vi "Test-DotNet-sendLaunchJob.vi"() -> ()   [LabVIEW 2013, in "EC1000-control.lvlib" / "SM1000-control.lvclass"]
uses:
  SM1000-control.lvclass
  DOTNET-settings.ctl
  Device-identification.ctl
  TCP-settings.ctl
panel:
  out "Ready":bool
  out "Job data":string
  out "Elapsed time":dbl caption="Elapsed time [ms]" format="%.2f"
  in  "Abort":bool
  out "Job busy":bool
  in  "Start job":bool
  in  "TCP settings":T1={"Target IP"="128.178.146.163", "Target TCP port"=12500, "TCP read mode"=enum."CRLF", "TCP read buffer"=4096, "Read timeout"=5000}
  in  "Job file path (.xml)":path=path "C:/LabVIEW/TJ-TransferJobs/SampleTestJobs/SM1000-Sim07.xml"
  in  "Device index":i32
  in  "DOTNET settings":T2={"Target IP"="128.178.146.163", "Target broadcast port"=11000, "Target communication port"=12200, "clientID"=-1, "Broadcast IP"="224.168.100.2", "Servercount"=-1, "Device IDs"=[{"Name"="EC1000", "IP"="128.178.146.163", "Mac address"="mac"}]}
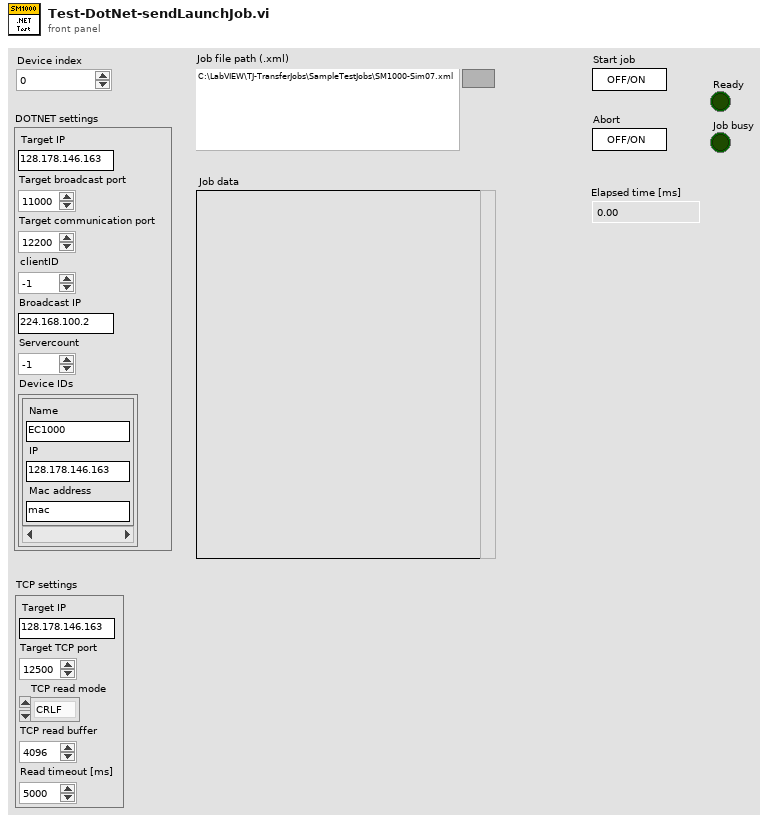
[diagram p1: front panel]
types:
  T1 = typedef "EC1000-control.lvlib/SM1000-control.lvclass/TCP-settings.ctl" = cluster{"Target IP":string, "Target TCP port":u16, "TCP read mode":enum16{"Standard", "Buffered", "CRLF", "Immediate"}, "TCP read buffer":i32, "Read timeout":i32}
  T2 = typedef "EC1000-control.lvlib/SM1000-control.lvclass/DOTNET-settings.ctl" = cluster{"Target IP":string, "Target broadcast port":i32, "Target communication port":i32, "clientID":i32, "Broadcast IP":string, "Servercount":i32, "Device IDs":T3[]}
  T3 = typedef "EC1000-control.lvlib/SM1000-control.lvclass/Device-identification.ctl" = cluster{"Name":string, "IP":string, "Mac address":string}
  T4 = typedef "EC1000-control.lvlib/SM1000-control.lvclass/Object-reference.ctl" = refnum<data-value>
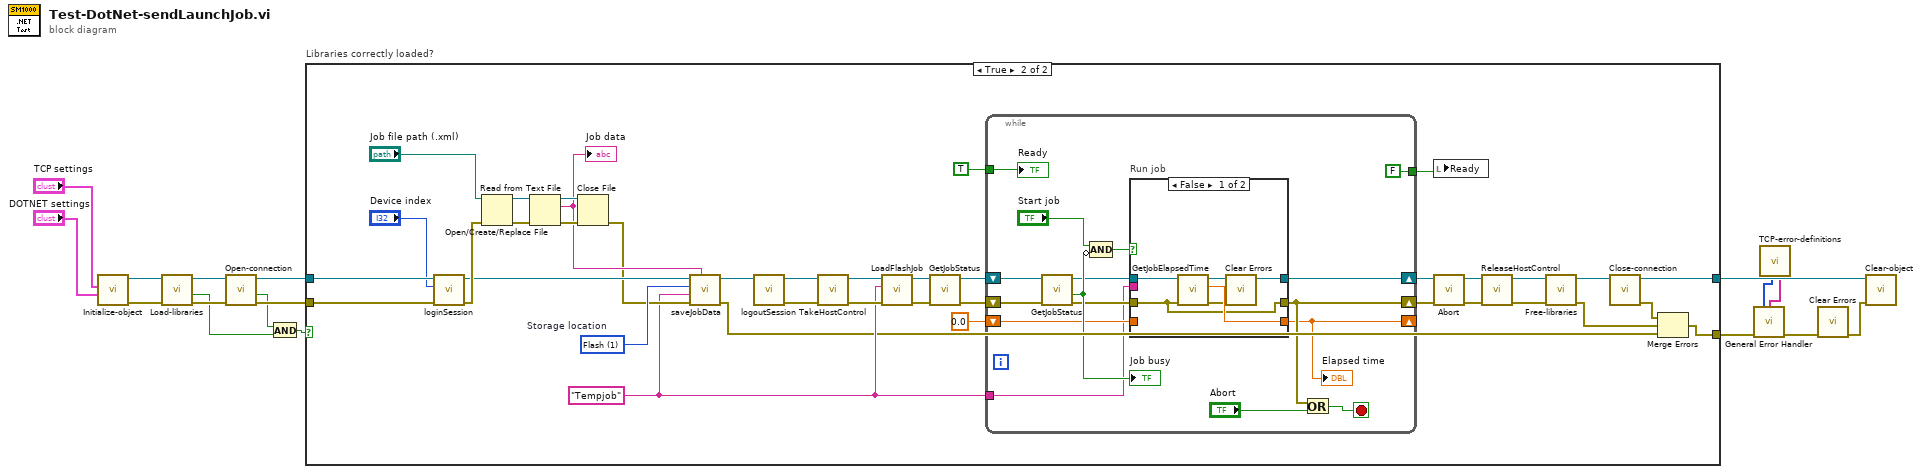
[diagram p0: block diagram]
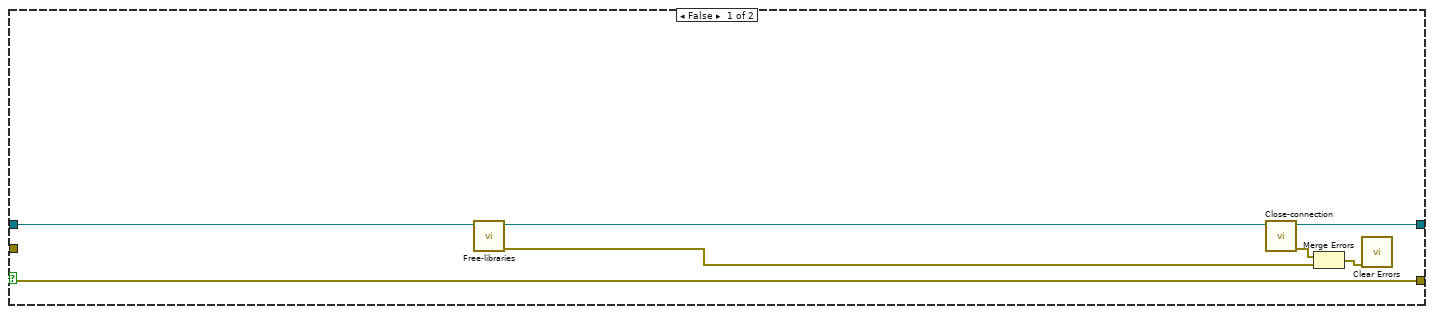
[diagram p2: hidden frame]
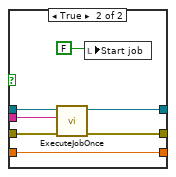
[diagram p3: hidden frame]
diagram:
  n1 = call "Initialize-object.vi"("DOTNET settings"="DOTNET settings", "TCP settings"="TCP settings") -> ("error out"=w15:errorcluster, "SM1000-control out"=w16:T4)  [unwired: 8 in]
  n2 = call "Load-libraries.vi"("error in (no error)"=w15, "SM1000-control in"=w16) -> ("error out"=w6:errorcluster, "Loaded?"=w3:bool, "SM1000-control out"=w9:T4)  [unwired: 7 in]
  n3 = call "Open-connection.vi"("error in (no error)"=w6, "SM1000-control in"=w9) -> ("error out"=w7:errorcluster, "Connected?"=w4:bool, "SM1000-control out"=w8:T4)  [unwired: 7 in]
  n4 = And(x=w4, y=w3) -> (x .and. y?=w5:bool)
  n5 = case "Libraries correctly loaded?" shown="True" w5 {
    tunnel: w8 -> [w23 w60]
    tunnel: w7 -> [w24 w59]
    tunnel: [w24 w61] -> w13
    tunnel: [w20 w44] -> w11
    frame False {
      n6 = call "Free-libraries.vi"("SM1000-control in"=w23) -> ("error out"=w22:errorcluster, "SM1000-control out"=w21:T4)  [unwired: 8 in, 1 out]
      n7 = call "Close-connection.vi"("SM1000-control in"=w21) -> ("error out"=w18:errorcluster, "SM1000-control out"=w20:T4)  [unwired: 8 in, 1 out]
      n8 = Merge Errors(w18, w22) -> (w19:errorcluster)
      n9 = call <vilib>:"Clear Errors.vi"("error in (no error)"=w19) -> ()  [unwired: 6 in, 1 out]
    }
    frame True {
      w50 = u16 1 items=["Flash"=1, "USB"=2]  # Storage location
      w32 = "Tempjob"
      n10 = call "loginSession.vi"("error in (no error)"=w59, "Device index"="Device index", "SM1000-control in"=w60) -> ("error out"=w52:errorcluster, "SM1000-control out"=w51:T4)  [unwired: 7 in]
      n11 = Open/Create/Replace File(file path (use dialog)="Job file path (.xml)", error in=w52) -> (refnum out=w54:refnum<file>, error out=w57:errorcluster)  [unwired: 4 in, 1 out]
      n12 = Read from Text File(file (use dialog)=w54, error in=w57) -> (refnum out=w55:refnum<file>, text=w49:string, error out=w56:errorcluster)  [unwired: 2 in, 1 out]
      "Job data" <- w49
      n13 = Close File(refnum=w55, error in=w56) -> (error out=w48:errorcluster)  [unwired: 1 out]
      n14 = call "saveJobData.vi"("Job data xml"=w49, "error in (no error)"=w48, "File name wo extension"=w32, "Storage location"=w50, "SM1000-control in"=w51) -> ("error out"=w26:errorcluster, "SM1000-control out"=w47:T4)  [unwired: 5 in]
      n15 = call "logoutSession.vi"("SM1000-control in"=w47) -> ("error out"=w42:errorcluster, "SM1000-control out"=w43:T4)  [unwired: 9 in]
      n16 = call "TakeHostControl.vi"("error in (no error)"=w42, "SM1000-control in"=w43) -> ("error out"=w38:errorcluster, "SM1000-control out"=w39:T4)  [unwired: 8 in]
      n17 = call "LoadFlashJob.vi"("error in (no error)"=w38, "Job name wo extension"=w32, "SM1000-control in"=w39) -> ("error out"=w36:errorcluster, "SM1000-control out"=w37:T4)  [unwired: 7 in]
      n18 = call "GetJobStatus.vi"("error in (no error)"=w36, "SM1000-control in"=w37) -> ("error out"=w35:errorcluster, "SM1000-control out"=w34:T4)  [unwired: 7 in, 1 out]
      n19 = while {
        shift-right: [w70] -> w30
        shift-left: w35 -> [w77]
        shift-right: [w69] -> w31
        shift-left: w34 -> [w78]
        shift-right: [w66] -> _
        shift-left: 0.0 ("Elapsed time") -> [w67]
        tunnel: w32 -> [w65]
        tunnel: TRUE -> [w64]
        tunnel: [FALSE] -> w25
        stop <- w72 stop-if-true
        n20 = call "GetJobStatus.vi"("error in (no error)"=w77, "SM1000-control in"=w78) -> ("error out"=w71:errorcluster, "Busy?"=w74:bool, "SM1000-control out"=w68:T4)  [unwired: 7 in]
        "Job busy" <- w74
        n21 = Compound Arithmetic op=AND("Start job", invert w74) -> (w75:bool)
        n22 = case "Run job" shown="False" w75 {
          tunnel: w71 -> [w79 w87]
          tunnel: [w79 w86] -> w70
          tunnel: [w83 w85] -> w69
          tunnel: w68 -> [w82 w88]
          tunnel: [w81 w90] -> w66
          tunnel: w67 -> [_ w90]
          tunnel: w65 -> [_ w89]
          frame False {
            n23 = call "GetJobElapsedTime.vi"("error in (no error)"=w79, "SM1000-control in"=w82) -> ("error out"=w80:errorcluster, "Elapsed time"=w81:dbl, "SM1000-control out"=w83:T4)  [unwired: 7 in]
            n24 = call <vilib>:"Clear Errors.vi"("error in (no error)"=w80) -> ()  [unwired: 6 in, 1 out]
          }
          frame True {
            n25 = call "ExecuteJobOnce.vi"("error in (no error)"=w87, "Job name wo extension"=w89, "SM1000-control in"=w88) -> ("error out"=w86:errorcluster, "SM1000-control out"=w85:T4)  [unwired: 7 in]
            n26 = local write "Start job"(FALSE) -> ()
          }
        }
        "Elapsed time" <- w66
        n27 = Or(x=w70, y="Abort") -> (x .or. y?=w72:bool)
        "Ready" <- w64
      }
      n28 = local write "Ready"(w25) -> ()
      n29 = call "Abort.vi"("error in (no error)"=w30, "SM1000-control in"=w31) -> ("error out"=w29:errorcluster, "SM1000-control out"=w28:T4)  [unwired: 8 in]
      n30 = call "ReleaseHostControl.vi"("error in (no error)"=w29, "SM1000-control in"=w28) -> ("error out"=w40:errorcluster, "SM1000-control out"=w41:T4)  [unwired: 8 in]
      n31 = call "Free-libraries.vi"("error in (no error)"=w40, "SM1000-control in"=w41) -> ("error out"=w62:errorcluster, "SM1000-control out"=w45:T4)  [unwired: 7 in, 1 out]
      n32 = call "Close-connection.vi"("SM1000-control in"=w45) -> ("error out"=w46:errorcluster, "SM1000-control out"=w44:T4)  [unwired: 8 in, 1 out]
      n33 = Merge Errors(w46, w62, w26) -> (w61:errorcluster)
    }
  }
  n34 = call "TCP-error-definitions.vi"() -> ("Descriptions"=w1:string[], "Error codes"=w2:i32[])  [unwired: 10 in]
  n35 = call <vilib>:"General Error Handler.vi"("[user-defined codes]"=w2, "[user-defined descriptions]"=w1, "error in (no error)"=w13) -> ("error out"=w14:errorcluster)  [unwired: 8 in, 4 out]
  n36 = call <vilib>:"Clear Errors.vi"("error in (no error)"=w14) -> ("error out"=w12:errorcluster)  [unwired: 6 in]
  n37 = call "Clear-object.vi"("error in (no error)"=w12, "SM1000-control"=w11) -> ()  [unwired: 8 in, 2 out]
